vi "Set Active Assert.vi"(8 "error in (no error)":errorcluster, 10 "Assert Name":string, 11 "Main Display in":refnum<class "Main Display.lvclass">) -> (0 "error out":errorcluster, 3 "Main Display out":refnum<class "Main Display.lvclass">)   [LabVIEW 2016, in "Assert API Components.lvlib" / "Assert Display.lvlib" / "Main Display.lvlib" / "Main Display.lvclass"]
uses:
  Main Display.lvclass
  Main Display.lvclass/Main Display.ctl
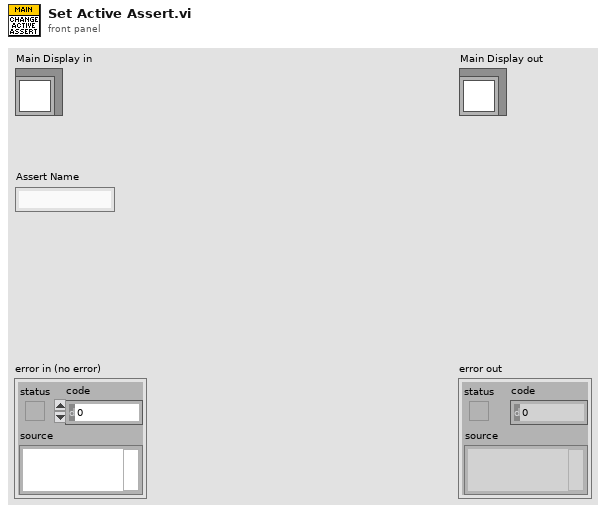
[diagram p1: front panel]
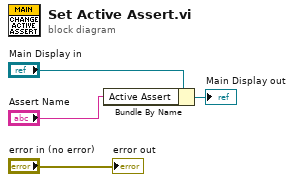
[diagram p0: block diagram]
diagram:
  n1 = Bundle By Name(cluster="Main Display in", "Active Assert"="Assert Name") -> (→"Main Display out":refnum<class "Main Display.lvclass">)
  "error out" <- "error in (no error)"
